vi "1-14.vi"() -> ()   [LabVIEW 2022 SP3]
panel:
  out "立方和":dbl
  in  "M":dbl
  in  "N":dbl
  out "数值":dbl
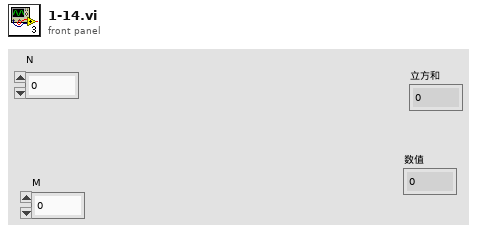
[diagram p1: front panel]
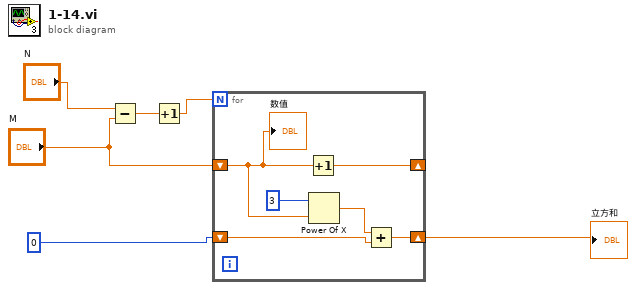
[diagram p0: block diagram]
diagram:
  n1 = Subtract(x="N", y="M") -> (x-y=w5:dbl)
  n2 = Increment(x=w5) -> (x+1=w4:dbl)
  n3 = for {
    N: w4 -> [_]
    shift-right: [w12] -> _
    shift-left: "M" -> [w10]
    shift-right: [w9] -> w2
    shift-left: 0 -> [w7]
    n4 = Increment(x=w10) -> (x+1=w12:dbl)
    n5 = Power Of X(1:w10, 2:3) -> (0:w8:dbl)
    n6 = Add(x=w8, y=w7) -> (x+y=w9:dbl)
    "数值" <- w10
  }
  "立方和" <- w2
